vi "Productos select.vi"(8 "error in (no error)":errorcluster, 10 "Producto":i32, 11 "Soda Actor in":refnum<class "Soda Actor.lvclass">) -> (0 "error out":errorcluster, 3 "Soda Actor out":refnum<class "Soda Actor.lvclass">)   [LabVIEW 2020, in "Soda Actor.lvlib" / "Soda Actor.lvclass"]
uses:
  Soda Actor.lvclass
  C:/Program Files/National Instruments/LabVIEW 2020/vi.lib/ActorFramework/Actor/Actor.lvclass
  <vilib>/ActorFramework/Actor/Actor.lvclass/Actor.ctl
  Soda Actor.lvclass/Soda Actor.ctl
  UI Actor Messages/Send product selection Msg/Send product selection Msg.lvclass/Send product selection Msg.ctl
  <vilib>/ActorFramework/Message Enqueuer/Message Enqueuer.lvclass/Message Enqueuer.ctl
  <vilib>/ActorFramework/Message Enqueuer/Enqueue.vi
  UI Actor Messages/Send product selection Msg/Send product selection Msg.lvclass
  C:/Program Files/National Instruments/LabVIEW 2020/vi.lib/ActorFramework/Message/Message.lvclass
  <vilib>/ActorFramework/Message Priority Queue/Priority Enqueue.vi
  <vilib>/ActorFramework/Actor/Actor.lvclass
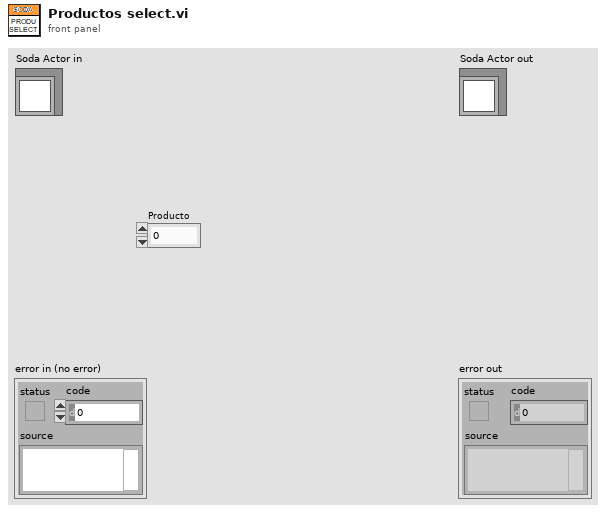
[diagram p1: front panel]
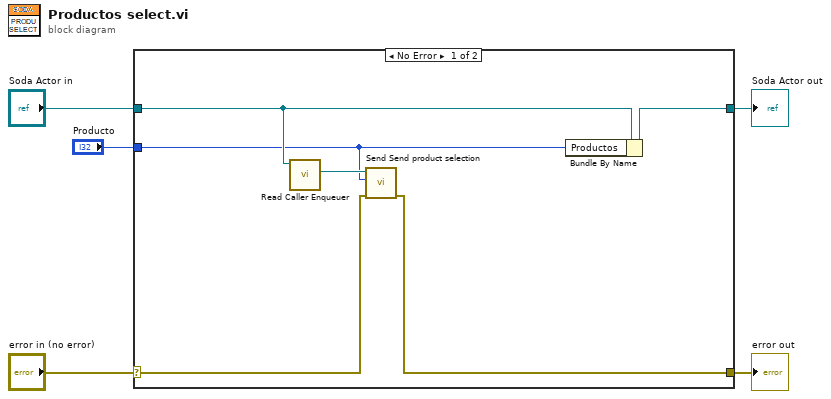
[diagram p0: block diagram]
diagram:
  n1 = case shown="No Error" "error in (no error)" {
    selector: "error in (no error)" -> [w7 w13]
    tunnel: [w6 w13] -> w4
    tunnel: [w11 w12] -> w2
    tunnel: "Soda Actor in" -> [w10 w12]
    tunnel: "Producto" -> [w8 _]
    frame No Error {
      n2 = call <vilib>:"Read Caller Enqueuer.vi"("Actor"=w10) -> ("Caller Enqueuer"=w9:refnum<class "Message Enqueuer.lvclass">)  [unwired: 10 in]
      n3 = call "Send Send product selection.vi"("error in (no error)"=w7, "Producto bueno"=w8, "Message Enqueuer"=w9) -> ("error out"=w6:errorcluster)  [unwired: 7 in, 1 out]
      n4 = Bundle By Name(cluster=w10, "Productos"=w8) -> (w11:refnum<class "Soda Actor.lvclass">)
    }
    frame Error {
    }
  }
  "error out" <- w4
  "Soda Actor out" <- w2
